vi "Pretrigger Buffer.vi"(5 "Mode":enum16{"Initialize", "Add", "Read"}(ring), 6 "Pretrigger Buffer Ref":refnum<vi>, 7 "Pretrigger Length":i32, 8 "# Channels":i32, 10 "New Data":sgl[](array[numeric])) -> (0 "Current Size":i32, 2 "Pretrigger Data":sgl[][](array[numeric]))   [LabVIEW 2019]
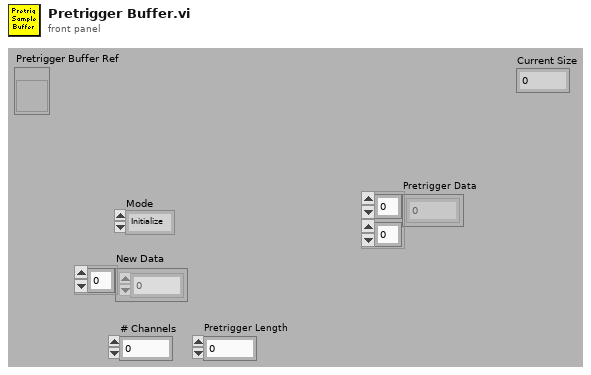
[diagram p1: front panel]
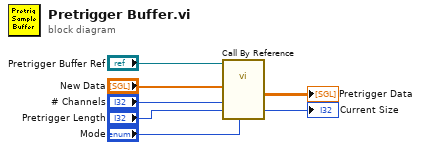
[diagram p0: block diagram]
diagram:
  n1 = call-by-ref "?"(reference="Pretrigger Buffer Ref", "Mode"="Mode", "Pretrigger Length"="Pretrigger Length", "# Channels"="# Channels", "New Data"="New Data") -> ("Current Size"=→"Current Size":i32, "Pretrigger Data"=→"Pretrigger Data":sgl[][])  [unwired: 6 in, 2 out]
